vi "Read Node Actor 1st CMD.vi"(8 "error in (no error)":errorcluster, 11 "Node Actor MSG in":refnum<class "Node Actor MSG.lvclass">) -> (0 "error out":errorcluster, 2 "Node Actor 1st CMD":T1 caption="Enum 3", 3 "Node Actor MSG out":refnum<class "Node Actor MSG.lvclass">)   [LabVIEW 2024, in "Node Actor MSG.lvclass"]
uses:
  Node Actor MSG.lvclass
  Node Actor MSG.lvclass/Node Actor MSG.ctl
  Type Def/Node Actor 1st CMD.ctl
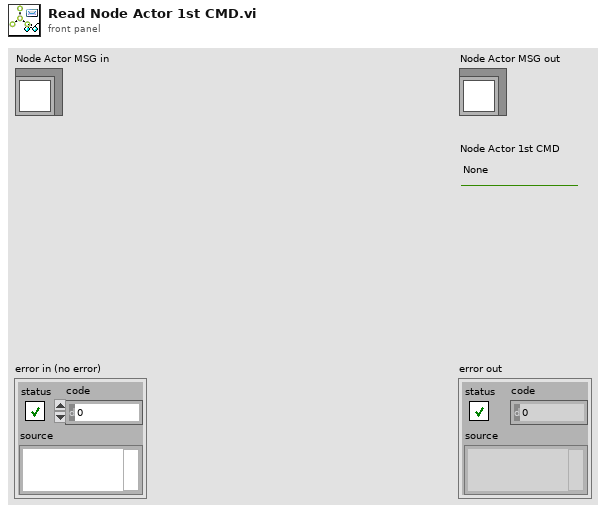
[diagram p1: front panel]
types:
  T1 = typedef "Node Actor 1st CMD.ctl" = enum16{"None", "Forward Message"}
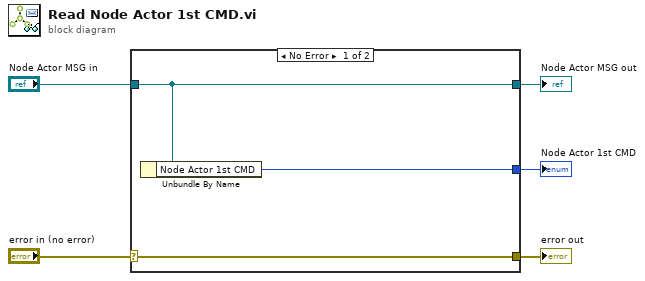
[diagram p0: block diagram]
diagram:
  n1 = case shown="No Error" "error in (no error)" {
    selector: "error in (no error)" -> [w8 w9]
    tunnel: [w8 w9] -> w4
    tunnel: [w7 w10] -> w2
    tunnel: "Node Actor MSG in" -> [w7 w10]
    tunnel: [w6 _] -> w1
    frame No Error {
      n2 = Unbundle By Name(w7) -> ("Node Actor 1st CMD"=w6:T1)
    }
    frame Error {
    }
  }
  "error out" <- w4
  "Node Actor MSG out" <- w2
  "Node Actor 1st CMD" <- w1
